vi "Save CID File.vi"(8 "error in (no error)":errorcluster, 9 "Content":string, 10 "File Name":string, 11 "Master Controller in":refnum<class "Master Controller.lvclass">) -> (0 "error out":errorcluster, 3 "Master Controller out":refnum<class "Master Controller.lvclass">)   [LabVIEW 2015, in "Master Controller Core.lvlib" / "Master Controller.lvclass"]
uses:
  Master Controller.lvclass
  <vilib>/ActorFramework/Actor/Actor.lvclass/Actor.ctl
  <vilib>/ActorFramework/Message Enqueuer/Message Enqueuer.lvclass/Message Enqueuer.ctl
  Master Controller.lvclass/Master Controller.ctl
  Master Controller Messages/EMS CID File Received Msg/EMS CID File Received Msg.lvclass/EMS CID File Received Msg.ctl
  <vilib>/ActorFramework/Message Enqueuer/Init from Existing Queue.vi
  <vilib>/ActorFramework/Message Enqueuer/Enqueue.vi
  <vilib>/ActorFramework/Message Priority Queue/Priority Enqueue.vi
  <vilib>/ActorFramework/Message Enqueuer/Message Enqueuer.lvclass
  Master Controller Messages/EMS CID File Received Msg/EMS CID File Received Msg.lvclass
  <vilib>/ActorFramework/Actor/Actor.lvclass
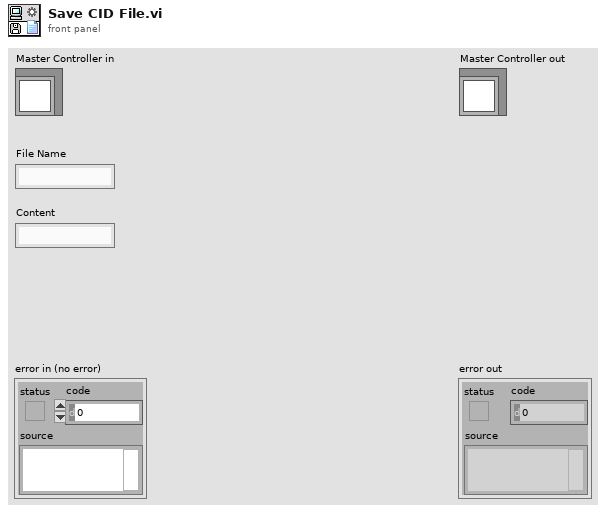
[diagram p1: front panel]
types:
  T1 = enum16{"open", "replace", "create", "open or create", "replace or create", "replace or create with confirmation"}
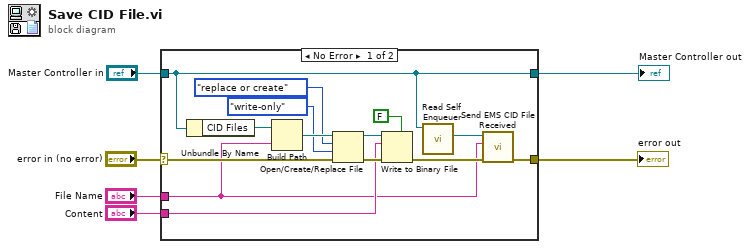
[diagram p0: block diagram]
diagram:
  n1 = case shown="No Error" "error in (no error)" {
    selector: "error in (no error)" -> [w17 w22]
    tunnel: [w8 w22] -> w5
    tunnel: [w11 w21] -> w3
    tunnel: "Master Controller in" -> [w11 w21]
    tunnel: "File Name" -> [w7 _]
    tunnel: "Content" -> [w13 _]
    frame No Error {
      n2 = Unbundle By Name(w11) -> ("CID Files"=w20:path)
      n3 = Build Path(base path=w20, name or relative path=w7) -> (appended path=w19:path)
      n4 = Open/Create/Replace File(file path (use dialog)=w19, error in=w17, operation (0:open)=T1."replace or create", access (0:read/write)=enum16{"read/write", "read-only", "write-only"}."write-only") -> (refnum out=w15:refnum<file>, error out=w14:errorcluster)  [unwired: 2 in, 1 out]
      n5 = Write to Binary File(file (use dialog)=w15, data=w13, error in=w14, 5:FALSE ("prepend array or string size? (T)")) -> (error out=w9:errorcluster)  [unwired: 2 in, 2 out]
      n6 = call <vilib>:"Read Self Enqueuer.vi"("Actor"=w11) -> ("Self Enqueuer"=w10:refnum<class "Message Enqueuer.lvclass">)  [unwired: 10 in]
      n7 = call "Send EMS CID File Received.vi"("error in (no error)"=w9, "File Name"=w7, "Message Enqueuer"=w10) -> ("error out"=w8:errorcluster)  [unwired: 7 in, 1 out]
    }
    frame Error {
    }
  }
  "error out" <- w5
  "Master Controller out" <- w3
